vi "GUI_Capillary_Transverse_Diagnostics.vi"() -> ()   [LabVIEW 2020]
uses:
  Shared/GUI_Template/GUI_master/tcp_new_data_event.ctl
  Shared/GUI_Template/GUI_master/tcp new data cluster.ctl
  General GUIs/Device GUIs/GUI_Cameras/color tables/image color table presets.ctl
  <vilib>/Platform/browser.llb/Open URL in Default Browser (string).vi
panel:
  in  "pos.Channel0::6":enum16{"1", "2", "3", "4", "5", "6"}(ring) caption="PL1-PMReflect-FW"
  in  "pos.Channel1::6":enum16{"1", "2", "3", "4", "5", "6"}(ring) caption="PL1-APLSideView FW"
  in  "GUIdevice 6":string="PL1-Filterwheels2"
  in  "Color table":T1=enum."Rainbow"
  in  "GUIdevice 5":string="PL1-SideSpec"
  out "Image::5":T2(plugin-control) caption="PL1-SideSpec"
  in  "GUIdevice 4":string="PL1-PMReflect"
  out "Image::4":T2(plugin-control) caption="PL1-PMReflect"
  in  "GUIdevice 3":string="PL1-SideView"
  out "Image::3":T2(plugin-control) caption="PL1-Sideview"
  in  "GUIdevice 2":string="PL1-APLSideview"
  out "Image::2":T2(plugin-control) caption="PL1-APLSideView"
  out "T/%  810 nm:":dbl
  out "T/%  656 nm:":dbl
  out "T/%  584 nm:":dbl
  out "T/%  532 nm:":dbl
  in  "pos.Channel2::1":enum16{"1", "2", "3", "4", "5", "6"}(ring) caption="PL1-SideSpec-FW"
  out "T/%  810 nm:":dbl
  out "T/%  656 nm:":dbl
  out "T/%  584 nm:":dbl
  out "T/%  532 nm:":dbl
  in  "calc filters":bool
  in  "pos.Channel0::1":enum16{"1", "2", "3", "4", "5", "6"}(ring) caption="PL1-SideView-FW"
  in  "Heater Alignment Directions":bool
  out "error IO 2":errorcluster
  out "tcp data event":T3
  in  "UDP error message":string
  in  "GUIdevice 1":string="PL1-FilterWheels"
  in  "stop":bool
  # "Capillary Monitoring Cameras"
  # "Filter Wheel Overview"
  # "Camera images"
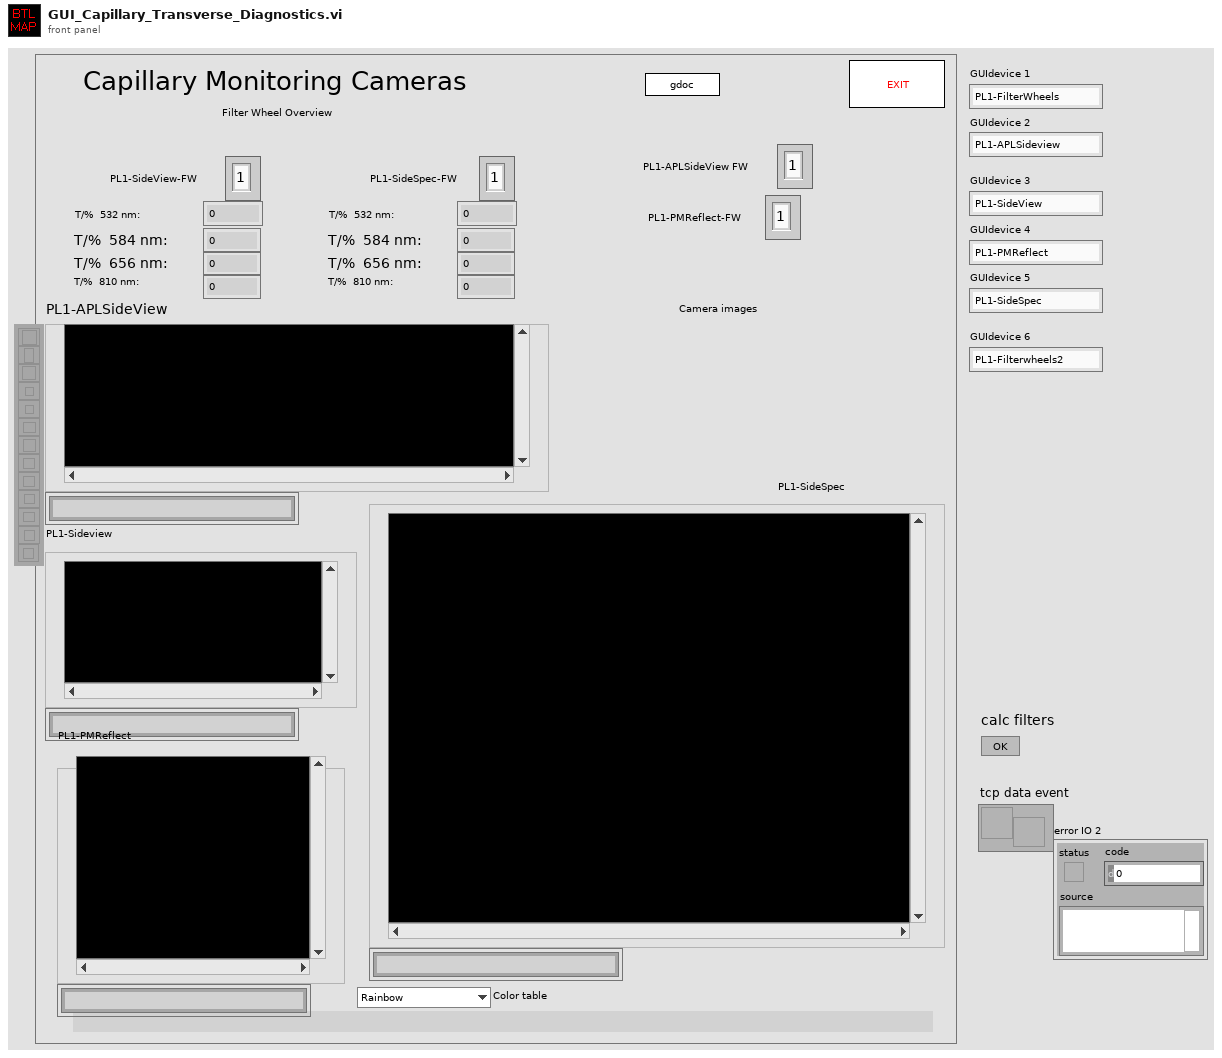
[diagram p1: front panel]
types:
  T1 = typedef "image color table presets.ctl" = enum16{"Greyscale", "Binary", "Gradient", "Rainbow", "Temperature", "enhance low", "blue yellow red", "BYR enhance low", "white blue yellow", "BWR enhance low", "make a new one"}
  T2 = typedef "IMAQ Image.ctl" = refnum<image>
  T3 = typedef "tcp_new_data_event.ctl" = refnum<user-event>
  T4 = typedef "Image Type" = u32
  T5 = typedef "tcp new data cluster.ctl" = cluster{"EventEnum":enum16{"new data", "connection status update"}, "Device name":string}
  T6 = enum32{"invalid app kind", "Development System", "Run Time System", "Student Edition", "Embedded LabVIEW", "Evaluation", "Custom"}
  T7 = enum32{"Invalid", "Standard", "Closed", "Hidden", "Minimized", "Maximized"}
  T8 = cluster{"Core":cluster{"Current VI Reference":refnum<vi>, "Close Panel on Exit?":bool}, "Heater timing offset":dbl, "Discharge timing offset":dbl, "Jet trigger":bool, "Tik1":u32, "Tik2":u32, "Fire Continues Allowed":bool}
  T9 = cluster{"Current VI Reference":refnum<vi>, "Close Panel on Exit?":bool}
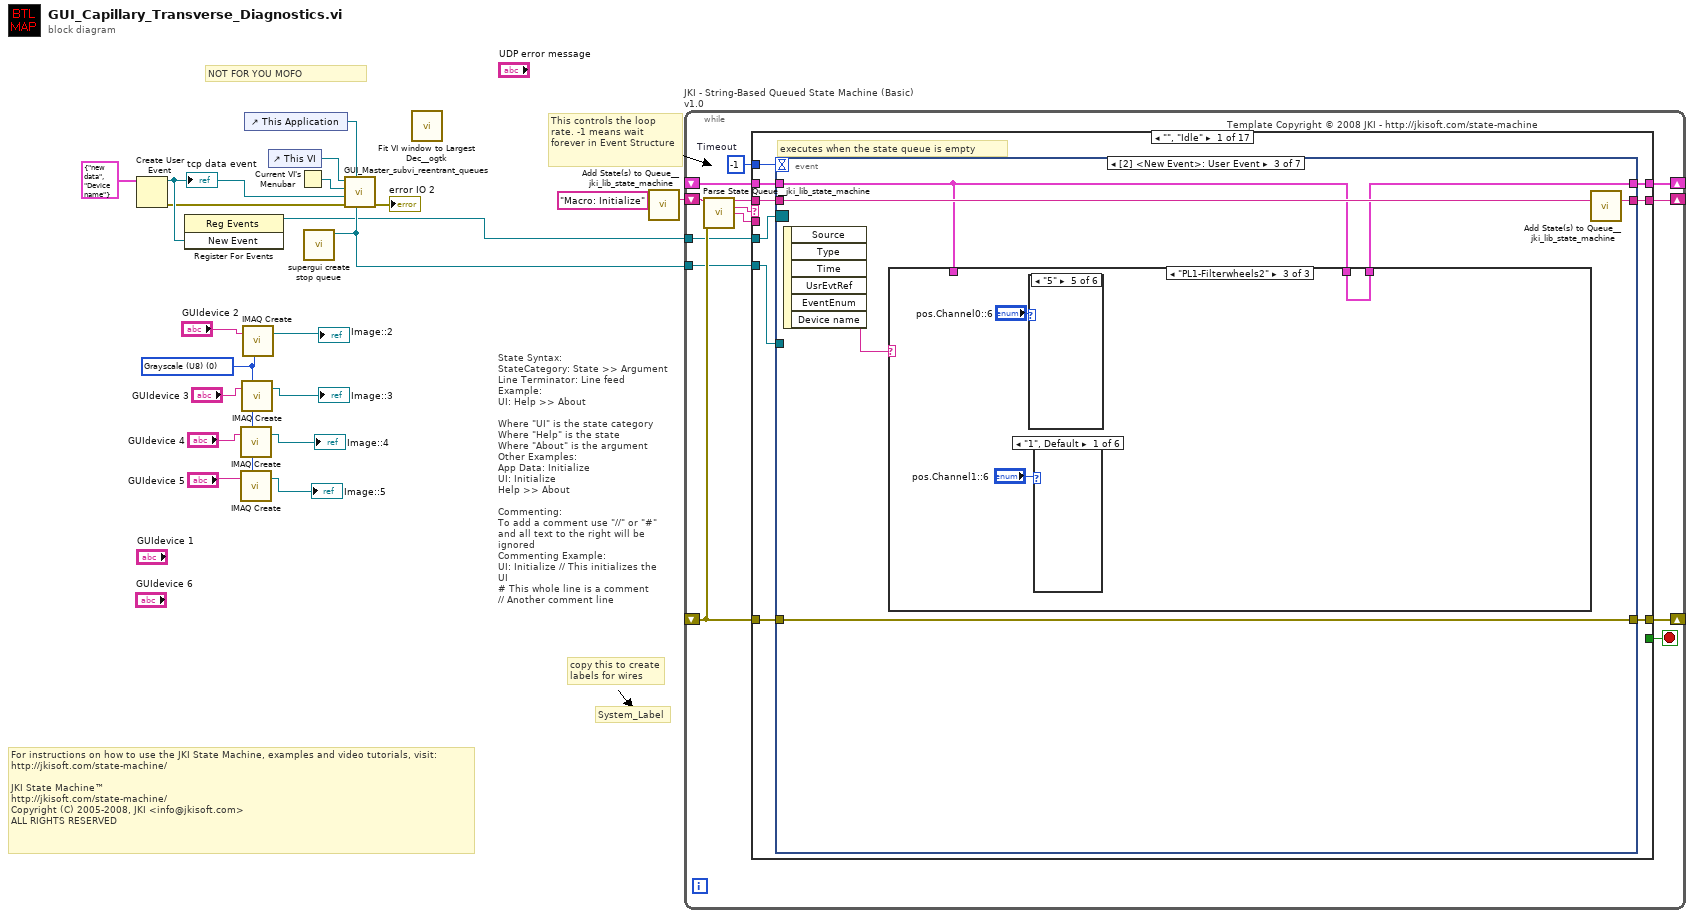
[diagram p0: block diagram]
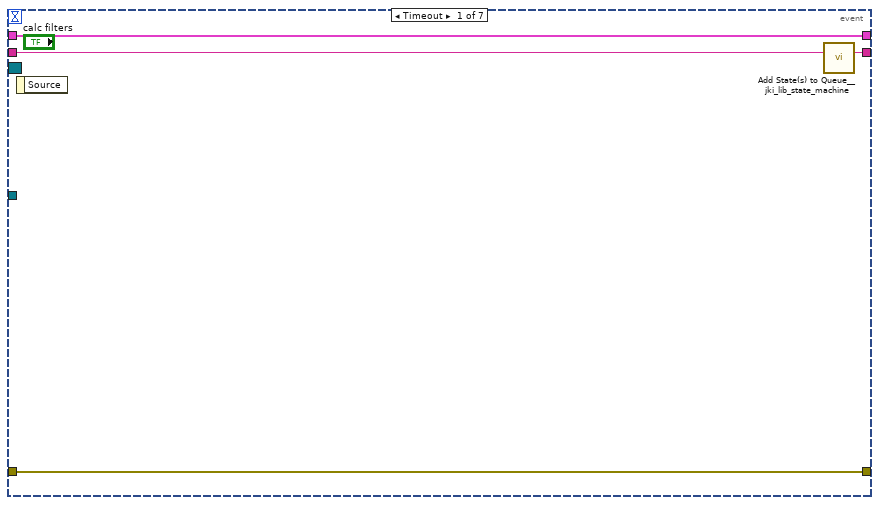
[diagram p2: hidden frame]
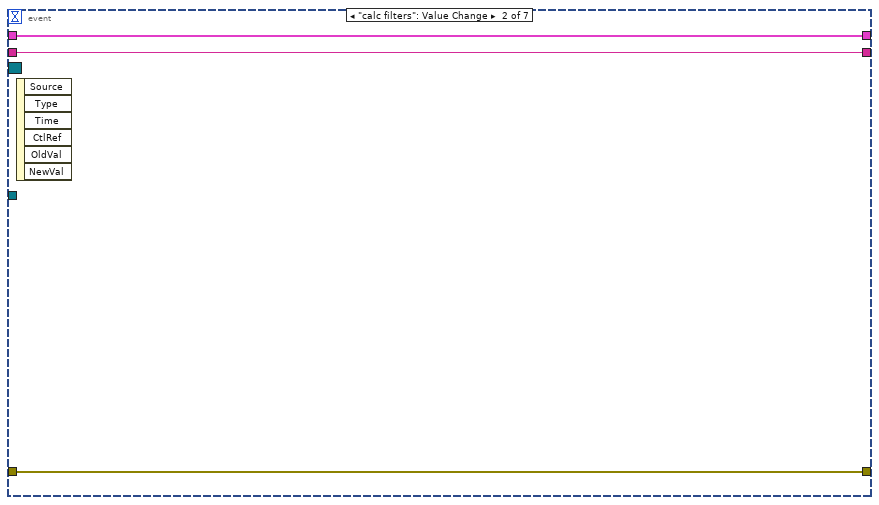
[diagram p3: hidden frame]
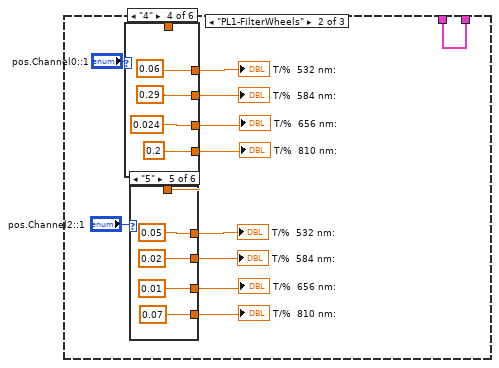
[diagram p5: hidden frame]
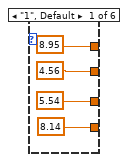
[diagram p6: hidden frame]
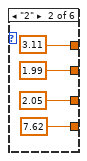
[diagram p7: hidden frame]
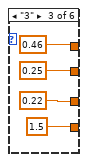
[diagram p8: hidden frame]
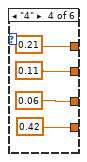
[diagram p9: hidden frame]
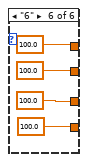
[diagram p10: hidden frame]
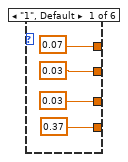
[diagram p11: hidden frame]
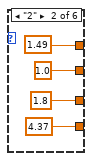
[diagram p12: hidden frame]
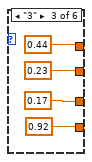
[diagram p13: hidden frame]
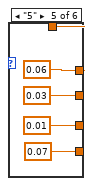
[diagram p14: hidden frame]
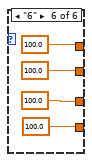
[diagram p15: hidden frame]
diagram:
  w5 = T4 0 items=["Grayscale (U8)", "Grayscale (I16)", "Grayscale (SGL)", "Complex (CSG)", "RGB (U32)", "HSL (U32)", "RGB (U64)", "Grayscale (U16)"] ("Image Type")
  # "For instructions on how to use the JKI State Machine, examples and video tutorials, visit:\nhttp://jkisoft.com/state-machine/\n\nJKI State Machine™\nhttp://jkisoft.com/state-machine/\nCopyright (C) 2005-2008, JKI <info@jkisoft.com>\nALL RIGHTS RESERVED"
  # "State Syntax:\nStateCategory: State >> Argument\nLine Terminator: Line feed\nExample:\nUI: Help >> About\n\nWhere \"UI\" is the state category\nWhere \"Help\" is the state\nWhere \"About\" is the argument\nOther Examples:\nApp Data: Initialize\nUI: Initialize\nHelp >> About\n\nCommenting:\nTo add a comment use \"//\" or \"#\" and all text to the right will be ignored\nCommenting Example:\nUI: Initialize // This initializes the UI\n# This whole line is a comment\n// Another comment line"
  # "copy this to create labels for wires"
  # "This controls the loop rate. -1 means wait forever in Event Structure"
  # "System_Label"
  # "NOT FOR YOU MOFO"
  n1 = Create User Event(user event datatype=T5 {"EventEnum"=enum."new data", "Device name"="Device name"} ("New Event")) -> (user event=w19:refnum<user-event>, error out=w18:errorcluster)  [unwired: 1 in]
  "tcp data event" <- w19
  n2 = register-events(w19) -> (reference out=w10:refnum<event-registration>)  [unwired: 2 in, 1 out]
  n3 = call "IMAQ Create"("Image Name"="GUIdevice 4", "Image Type"=w5) -> ("New Image"=→"Image::4":T2)  [unwired: 3 in, 1 out]
  n4 = call "IMAQ Create"("Image Name"="GUIdevice 5", "Image Type"=w5) -> ("New Image"=→"Image::5":T2)  [unwired: 3 in, 1 out]
  n5 = call "IMAQ Create"("Image Name"="GUIdevice 3", "Image Type"=w5) -> ("New Image"=→"Image::3":T2)  [unwired: 3 in, 1 out]
  n6 = call "IMAQ Create"("Image Name"="GUIdevice 2", "Image Type"=w5) -> ("New Image"=→"Image::2":T2)  [unwired: 3 in, 1 out]
  n7 = control-ref of="This Application"() -> (w20:refnum<vi>)
  n8 = control-ref of="This VI"() -> (w14:refnum<vi>)
  n9 = Current VI's Menubar() -> (w16:refnum<k9>)
  n10 = call "supergui create stop queue.vi"() -> ("STOP Queue out"=w11:refnum<queue>)  [unwired: 11 in]
  n11 = call "GUI_Master_subvi_reentrant_queues.vi"("STOP Queue in"=w11, "This Application"=w20, "error in (no error)"=w18, "tcp data event"=w19, "Caller menu reference"=w16, "Caller VI ref"=w14) -> ("error out"=→"error IO 2":errorcluster)  [unwired: 5 in]
  n12 = call <userlib>:"Fit VI window to Largest Dec__ogtk.vi"() -> ()  [unwired: 6 in, 2 out]
  n13 = call <vilib>:"Add State(s) to Queue__jki_lib_state_machine.vi"("State(s) in (\"\")"="Macro: Initialize") -> ("States Out"=w12:string)  [unwired: 14 in]
  n14 = while "JKI - String-Based Queued State Machine (Basic) v1.0" {
    shift-right: [w26] -> _
    shift-left: _ -> [w25]
    shift-right: [w29] -> _
    shift-left: _ -> [w23]
    shift-right: [w28] -> _
    shift-left: w12 -> [w30]
    tunnel: w10 -> [w22]
    tunnel: w11 -> [w21]
    stop <- w27 stop-if-true
    w24 = -1  # Timeout
    # "Template Copyright © 2008 JKI - http://jkisoft.com/state-machine"
    n15 = call <vilib>:"Parse State Queue__jki_lib_state_machine.vi"("State Queue"=w30, "Error In (no error)"=w23) -> ("Remaining States"=w32:string, "Current State"=w33:string, "Arguments"=w31:string)  [unwired: 11 in]
    n16 = case shown="\"\", \"Idle\"" w33 {
      selector: w33 -> [_ _ w171 _ _ _ _ _ _ _ _ _ _ _ _ _ _]
      tunnel: w32 -> [w42 w170 w175 w193 w199 w204 w208 w219 w225 w229 w235 w241 w252 w278 w283 w293 w297]
      tunnel: w31 -> [_ _ _ _ _ _ _ _ _ _ _ w236 w246 _ _ _ _]
      tunnel: w25 -> [w40 w167 w173 w184 w196 w202 w205 _ w220 w226 w233 w239 w248 w275 w280 w290 w294]
      tunnel: [w39 w168 w177 w190 errorcluster {"status"=FALSE, "code"=0, "source"=""} ("error out") w201 w206 w216 w221 w227 w232 w237 w249 w276 w281 w291 w295] -> w29
      tunnel: w23 -> [w38 w168 w176 w190 w195 w201 w206 w216 w222 w227 w232 w238 w250 w276 w281 w291 w295]
      tunnel: [w41 w169 w174 w192 w198 w203 w207 w218 w224 w228 w234 w240 w251 w277 w282 w292 w296] -> w28
      tunnel: [_ _ _ _ _ TRUE _ _ _ _ _ _ _ _ _ _ _] -> w27
      tunnel: [w34 w167 w173 w191 w196 w202 w205 w217 w220 w226 w233 w239 w248 w275 w280 w290 w294] -> w26
      tunnel: w24 -> [w37 _ _ _ _ _ _ _ _ _ _ _ _ _ _ _ _]
      tunnel: w22 -> [w36 _ _ _ _ _ _ _ _ _ _ _ _ _ _ _ _]
      tunnel: w21 -> [w35 _ _ _ _ _ _ _ _ _ _ _ _ _ _ _ _]
      frame "", "Idle" {
        # "executes when the state queue is empty"
        n17 = event shown="[2] <New Event>: User Event" {
          selector: w36 -> [_ _ _ _ _ _ _]
          dyn-events: _ -> [_ _ _ _ _ _ _]
          timeout: w37 -> [_ _ _ _ _ _ _]
          tunnel: w42 -> [w46 w48 w55 w130 w151 w156 w166]
          tunnel: [w45 w48 w54 w130 w150 w156 w165] -> w41
          tunnel: w40 -> [w43 w49 w51 w131 w148 w155 w163]
          tunnel: [w44 w47 w53 w119 w149 w153 w164] -> w39
          tunnel: w38 -> [w44 w47 w53 w120 w149 w154 w164]
          tunnel: [w43 w49 w50 w131 w148 w155 w163] -> w34
          tunnel: w35 -> [_ _ _ _ w145 _ _]
          event Timeout {
            n18 = event-data() -> ()  [unwired: 1 in, 1 out]
            n19 = call <vilib>:"Add State(s) to Queue__jki_lib_state_machine.vi"("State(s) in (\"\")"=w46) -> ("States Out"=w45:string)  [unwired: 14 in]
          }
          event "calc filters": Value Change {
            n20 = event-data() -> ()  [unwired: 1 in, 6 out]
          }
          event User Event {
            n21 = event-data() -> ("Device name"=w52:string)  [unwired: 1 in, 5 out]
            n22 = case shown="\"PL1-Filterwheels2\"" w52 {
              tunnel: w51 -> [_ _ _]
              tunnel: w51 -> [w56 w67 w118]
              tunnel: [w56 w67 w118] -> w50
              frame "False", Default {
              }
              frame "PL1-FilterWheels" {
                n23 = case shown="\"4\"" "pos.Channel0::1" {
                  tunnel: [_ _ _ _ w111 _] -> _
                  tunnel: [0.07 1.49 0.44 0.06 w111 100.0] -> w66
                  tunnel: [0.03 1.0 0.23 0.29 0.03 100.0] -> w65
                  tunnel: [0.03 1.8 0.17 0.024 0.01 100.0] -> w64
                  tunnel: [0.37 4.37 0.92 0.2 0.07 100.0] -> w63
                  frame "1", Default {
                  }
                  frame "2" {
                  }
                  frame "3" {
                  }
                  frame "4" {
                  }
                  frame "5" {
                    w111 = 0.06
                  }
                  frame "6" {
                  }
                }
                "T/%  532 nm:" <- w66
                "T/%  584 nm:" <- w65
                "T/%  656 nm:" <- w64
                "T/%  810 nm:" <- w63
                n24 = case shown="\"5\"" "pos.Channel2::1" {
                  tunnel: [_ _ _ _ w87 _] -> _
                  tunnel: [8.95 3.11 0.46 0.21 w87 100.0] -> w61
                  tunnel: [4.56 1.99 0.25 0.11 0.02 100.0] -> w60
                  tunnel: [5.54 2.05 0.22 0.06 0.01 100.0] -> w59
                  tunnel: [8.14 7.62 1.5 0.42 0.07 100.0] -> w58
                  frame "1", Default {
                  }
                  frame "2" {
                  }
                  frame "3" {
                  }
                  frame "4" {
                  }
                  frame "5" {
                    w87 = 0.05
                  }
                  frame "6" {
                  }
                }
                "T/%  532 nm:" <- w61
                "T/%  584 nm:" <- w60
                "T/%  656 nm:" <- w59
                "T/%  810 nm:" <- w58
              }
              frame "PL1-Filterwheels2" {
                n25 = case shown="\"5\"" "pos.Channel0::6" {
                  frame "1", Default {
                  }
                  frame "2" {
                  }
                  frame "3" {
                  }
                  frame "4" {
                  }
                  frame "5" {
                  }
                  frame "6" {
                  }
                }
                n26 = case shown="\"1\", Default" "pos.Channel1::6" {
                  frame "1", Default {
                  }
                  frame "2" {
                  }
                  frame "3" {
                  }
                  frame "4" {
                  }
                  frame "5" {
                  }
                  frame "6" {
                  }
                }
              }
            }
            n27 = call <vilib>:"Add State(s) to Queue__jki_lib_state_machine.vi"("State(s) in (\"\")"=w55) -> ("States Out"=w54:string)  [unwired: 14 in]
          }
          event Value Change {
            # "Chech whether user input for color table\nother than Ni pallete"
            # "When user cancels the make new one color table \nthen color table value changed to rainbow"
            n28 = event-data() -> ()  [unwired: 1 in, 6 out]
            n29 = control-ref of="Image::4"() -> (w121:refnum<vi>)
            n30 = property on="Color table" class="Enum (strict)"() -> ("Strings []"=w125:string[])  [unwired: 2 in, 2 out]
            n31 = Format Into String("Color table") -> (resulting string=w124:string)  [unwired: 3 in, 1 out]
            n32 = call "IMAQ color table presets.vi"("Color table"="Color table") -> ("Make new one cancelled"=w129:bool, "Array"=w122:cluster{"R":u8, "G":u8, "B":u8}[])  [unwired: 9 in]
            n33 = Search 1D Array(1D array=w125, element=w124) -> (index of element=w127:i32)  [unwired: 1 in]
            n34 = Greater Or Equal?(x=w127, y=5) -> (x >= y?=w126:bool)
            n35 = case shown="False" w126 {
              tunnel: w122 -> [_ w140]
              tunnel: "Color table" -> [w135 _]
              tunnel: w120 -> [w134 w137]
              tunnel: [w133 w139] -> w119
              tunnel: w129 -> [_ w138]
              tunnel: w121 -> [w132 w136]
              frame False {
                n36 = property on="Property Node" class="ImageControl"(reference=w132, error in=w134, "Palette Type"=w135) -> (error out=w133:errorcluster)  [unwired: 1 out]
              }
              frame True {
                w141 = u32 5 items=["Grayscale", "Binary", "Gradient", "Rainbow", "Temperature", "User Defined"] ("Palette:Palette Type")
                n37 = property on="Property Node" class="ImageControl"(reference=w136, error in=w137, "Palette Type"=w141, "User Palette"=w140) -> (error out=w139:errorcluster)  [unwired: 1 out]
                n38 = case shown="True" w138 {
                  tunnel: w137 -> [_ w142]
                  frame False {
                  }
                  frame True {
                    n39 = property on="Color table" class="Enum (strict)"(error in=w142, "Val(Sgnl)"=image_color_table_presets."Rainbow" ("Value (Signaling)")) -> ()  [unwired: 1 in, 2 out]
                  }
                }
              }
            }
          }
          event "stop": Value Change {
            # "Exit Button Value Change (pressed) Event\n(this executes Macro: Exit to terminate the VI)"
            n40 = event-data() -> ()  [unwired: 1 in, 6 out]
            n41 = Release Queue(queue=w145, force destroy? (F)=TRUE) -> (error out=w146:errorcluster)  [unwired: 1 in, 2 out]
            n42 = call <vilib>:"Clear Errors.vi"("error in (no error)"=w146) -> ()  [unwired: 5 in, 2 out]
            n43 = call <vilib>:"Add State(s) to Queue__jki_lib_state_machine.vi"("State(s) in Front (\"\")"="Macro: Exit", "State(s) in (\"\")"=w151) -> ("States Out"=w150:string)  [unwired: 13 in]
          }
          event "Heater Alignment Directions": Value Change {
            n44 = event-data() -> ()  [unwired: 1 in, 6 out]
            n45 = case shown="True" "Heater Alignment Directions" {
              tunnel: w154 -> [w157 w160]
              tunnel: [w157 w159] -> w153
              frame False {
              }
              frame True {
                n46 = call-poly <vilib>:"Open URL in Default Browser.vi"("error in (no error)"=w160, "URL"="https://docs.google.com/document/d/11rq5sV6otXhl_RvgO5tmtLmhp9iuGuESqiH9zh7F1jg/edit?usp=sharing") -> ("error out"=w159:errorcluster)  [unwired: 4 in, 1 out]
              }
            }
          }
          event Panel Close? {
            # "Discard the event because we'll close the front panel ourselves in Macro: Exit"
            # "Close Panel button (pressed) Event\n(this executes Macro: Exit to terminate the VI)"
            n47 = event-data() -> ()  [unwired: 1 in, 1 out]
            n48 = event-data("Discard?"=TRUE) -> ()  [unwired: 1 in, 1 out]
            n49 = call <vilib>:"Add State(s) to Queue__jki_lib_state_machine.vi"("State(s) in Front (\"\")"="Macro: Exit", "State(s) in (\"\")"=w166) -> ("States Out"=w165:string)  [unwired: 13 in]
          }
        }
      }
      frame "---------- Core ----------" {
        # "Do not put any code in this frame.\n(it is a separator no-op)"
        n50 = call <vilib>:"Add State(s) to Queue__jki_lib_state_machine.vi"("State(s) in (\"\")"=w170) -> ("States Out"=w169:string)  [unwired: 14 in]
      }
      frame Default {
        w180 = 42 items=["No error", "Argument error", "Memory is full", "Out of zone", "End of file", "File already open", "Generic file I/O error", "File not found", "File permission error", "Disk is full", "Duplicate path", "Too many files open", "System feature not enabled", "Resource file not found", "Cannot add resource", "Resource not found", "Image not found", "Image memory error", "Pen does not exist", "Config type invalid", "Config token not found", "Config parse error", "Config memory error", "Bad external code format", "Bad external code offset", "External code not present", "Null window", "Destroy window error", "Null menu", "Print aborted", "Bad print record", "Print driver error", "Windows error during printing", "Memory error during printing", "Print dialog error", "Generic print error", "Invalid device refnum", "Device not found", "Device parameter error", "Device unit error", "Cannot open device", "Device call aborted", "Generic error", "Cancelled by user", "Object ID too low", "Object ID too high", "Object not in heap", "Unknown heap", "Unknown object (invalid DefProc)", "Unknown object (DefProc not in table)", "Message out of range", "Invalid (null) method", "Unknown message", "Manager call not supported", "Bad address", "Network operation in progress", "Network operation timed out", "Connection is busy", "Network attribute not supported", "Network error", "Address in use", "System out of memory", "Connection aborted", "Connection refused", "Not connected", "Already connected", "Connection closed", "Initialization error (interapplication manager)", "Bad occurrence", "Wait on unbound occurrence handler", "Occurrence queue overflow", "Datalog type conflict", "Unused", "Unrecognized type (interapplication manager)", "Memory corrupt", "Failed to make temporary DLL", "Old CIN version", "Drag socket not found", "Failed to load drop-object", "Failed to register OLE object", "Failed to release OLE object", "Format specifier type mismatch", "Unknown format specifier", "Too few format specifiers", "Too many format specifiers", "Scan failed", "Newer CIN version", "Error converting to variant", "Runtime menu error", "Password tampered", "Variant attribute not found", "Incompatible variant data type", "Event data is not available", "Event Store is not present", "Occurrence is not found", "Event Queue is not created", "Event info is not available", "Refnum passed is NULL", "Error retrieving Class GUID", "Error retrieving CoClass GUID", "Error retrieving TypeLib GUID.", "Bad built application magic bytes.", "Specific driver is different from the specific driver associated with the Logical Name.", "There is no session opened to the class driver.", "Max Error", "MAX - Error with config objects", "MAX - Error loading configuration", "MAX - Group not supported"]
        # "Current State"
        # "Do not delete, rename, or modify this frame.\n(this is used to capture unhandled states and typos)"
        # "Handle mistyped state name (developer tool)"
        n51 = Format Into String(format string="Software Exception: Unhandled State \"%s\"." ("message"), error in=w176, w171) -> (resulting string=w179:string, error out=w178:errorcluster)  [unwired: 1 in]
        n52 = call <vilib>:"Error Cluster From Error Code.vi"("show call chain? (False)"=TRUE, "error in (no error)"=w178, "error message (\"\")"=w179, "error code (0)"=w180) -> ("error out"=w177:errorcluster)  [unwired: 5 in]
        n53 = call <vilib>:"Add State(s) to Queue__jki_lib_state_machine.vi"("State(s) in (\"\")"=w175) -> ("States Out"=w174:string)  [unwired: 14 in]
      }
      frame "Initialize Core Data" {
        # "Do not delete, rename, or modify this frame.\n(this is used to determine panel behavior on exit)"
        # "originally closed?"
        # "exe?"
        # "If panel starts closed or is an EXE, then close it when we exit"
        n54 = property class="VI"() -> ("Front Panel.Open"=w189:bool)  [unwired: 2 in, 2 out]
        n55 = property class="App"() -> ("App.Kind"=w188:T6)  [unwired: 2 in, 2 out]
        n56 = control-ref of="Current VI Reference"() -> (w182:refnum<vi>)
        n57 = Not(x=w189) -> (.not. x?=w186:bool)
        n58 = Equal?(x=w188, y=T6."Run Time System" ("Application:Kind")) -> (x = y?=w185:bool)
        n59 = Or(x=w186, y=w185) -> (x .or. y?=w183:bool)
        n60 = Bundle By Name(cluster=w184, "Core.Current VI Reference"=w182, "Core.Close Panel on Exit?"=w183) -> (w191:T8)
        n61 = call <vilib>:"Add State(s) to Queue__jki_lib_state_machine.vi"("State(s) in (\"\")"=w193) -> ("States Out"=w192:string)  [unwired: 14 in]
      }
      frame "Error Handler" {
        # "Unhandled Error -- Display it"
        # "Handle any errors here.\nYou can also output any states to clean-up after errors occur"
        # "Clear error"
        n62 = call <vilib>:"General Error Handler.vi"("error in (no error)"=w195) -> ()  [unwired: 10 in, 5 out]
        n63 = call <vilib>:"Add State(s) to Queue__jki_lib_state_machine.vi"("State(s) in Front (\"\")"="/* Post Error States", "State(s) in (\"\")"=w199) -> ("States Out"=w198:string)  [unwired: 13 in]
      }
      frame "Exit" {
        # "Do not put any code in this frame.\n(No errors that occur here will be handled.)"
        n64 = call <vilib>:"Add State(s) to Queue__jki_lib_state_machine.vi"("State(s) in (\"\")"=w204) -> ("States Out"=w203:string)  [unwired: 14 in]
      }
      frame "---------- Data ----------" {
        # "Do not put any code in this frame.\n(It is a separator no-op. You can make a copy of this frame to create a new Data frame)"
        n65 = call <vilib>:"Add State(s) to Queue__jki_lib_state_machine.vi"("State(s) in (\"\")"=w208) -> ("States Out"=w207:string)  [unwired: 14 in]
      }
      frame "Data: Initialize" {
        w209 = FALSE  # Fire Continues Allowed
        w211 = u32 0  # Tik1
        w210 = u32 0  # Tik2
        w212 = FALSE  # Jet trigger
        w213 = 0.0  # Discharge timing offset
        w214 = 0.0  # Heater timing offset
        w215 = T9 {"Current VI Reference"=refnum, "Close Panel on Exit?"=FALSE}  # Core
        # "do not delete - used by framework"
        # "Expand Bundle to add new data elements to shift register data."
        # "Add new data here."
        # "Data names and types of shift register data are defined by this bundle."
        # "Initialize the shift-register data, here.\n(data names are defined by what you wire into the bundle function)"
        n66 = Bundle("Core"=w215, "Heater timing offset"=w214, "Discharge timing offset"=w213, "Jet trigger"=w212, "Tik1"=w211, "Tik2"=w210, "Fire Continues Allowed"=w209) -> (w217:T8)  [unwired: 1 in]
        n67 = call <vilib>:"Add State(s) to Queue__jki_lib_state_machine.vi"("State(s) in (\"\")"=w219) -> ("States Out"=w218:string)  [unwired: 14 in]
      }
      frame "Data: Cleanup" {
        # "Cleanup any data and references, here.\n(this is called automatically, by the Macro: Exit)"
        n68 = Unbundle By Name(w220) -> ("Core.Current VI Reference"=w223:refnum<vi>)
        n69 = Close Reference(reference=w223, error in (no error)=w222) -> (error out=w221:errorcluster)
        n70 = call <vilib>:"Add State(s) to Queue__jki_lib_state_machine.vi"("State(s) in (\"\")"=w225) -> ("States Out"=w224:string)  [unwired: 14 in]
      }
      frame "---------- UI ----------" {
        # "Do not put any code in this frame.\n(It is a separator no-op. You can make a copy of this frame to create a new UI frame)"
        n71 = call <vilib>:"Add State(s) to Queue__jki_lib_state_machine.vi"("State(s) in (\"\")"=w229) -> ("States Out"=w228:string)  [unwired: 14 in]
      }
      frame "UI: Initialize" {
        # "Initialize the User Interface, here.\n(this is called automatically, by the Macro: Init)"
        n72 = control-ref of="Color table"() -> (w230:refnum<vi>)
        n73 = property on="Property Node" class="Enum (strict)"(reference=w230, "Value"=image_color_table_presets."Rainbow" ("Color table")) -> ()  [unwired: 1 in, 2 out]
        n74 = call <vilib>:"Add State(s) to Queue__jki_lib_state_machine.vi"("State(s) in (\"\")"=w235) -> ("States Out"=w234:string)  [unwired: 14 in]
      }
      frame "UI: Cursor Set" {
        # "Argument"
        # "Set and Unset Cursor Busy.\n(Usage: \"UI: Cursor Set >> Busy|Idle\")"
        n75 = case shown="\"Idle\", Default" w236 {
          tunnel: w238 -> [w243 w245]
          tunnel: [w242 w244] -> w237
          frame "Idle", Default {
            n76 = call <vilib>:"Unset Busy.vi"("error in (no error)"=w243) -> ("error out"=w242:errorcluster)  [unwired: 10 in]
          }
          frame "Busy" {
            n77 = call <vilib>:"Set Busy.vi"("error in (no error)"=w245) -> ("error out"=w244:errorcluster)  [unwired: 9 in, 1 out]
          }
        }
        n78 = call <vilib>:"Add State(s) to Queue__jki_lib_state_machine.vi"("State(s) in (\"\")"=w241) -> ("States Out"=w240:string)  [unwired: 14 in]
      }
      frame "UI: Front Panel State" {
        # "Argument"
        # "Set Front Panel Open or Closed\n(Usage: \"UI: Front Panel State >> Open|Close\")"
        n79 = Unbundle By Name(w248) -> ("Core.Current VI Reference"=w247:refnum<vi>)
        n80 = case shown="\"Close\"" w246 {
          tunnel: w250 -> [w256 w269]
          tunnel: [w258 w270] -> w249
          tunnel: w247 -> [w257 w267]
          frame "Open", Default {
            n81 = property class="VI"(reference=w257, error in=w256) -> (reference out=w254:refnum<vi>, error out=w255:errorcluster, "Front Panel.Open"=w253:bool)
            n82 = case shown="False" w253 {
              tunnel: [w261 w264] -> w258
              tunnel: w255 -> [w260 w264]
              tunnel: w254 -> [w259 _]
              frame False {
                n83 = invoke class="VI" method="FP.Open"(reference=w259, error in=w260, "Activate"=TRUE, "State"=T7."Standard") -> (error out=w261:errorcluster)  [unwired: 1 in, 4 out]
              }
              frame True {
              }
            }
          }
          frame "Close" {
            n84 = property class="VI"(reference=w267, error in=w269) -> (reference out=w266:refnum<vi>, error out=w268:errorcluster, "Front Panel.Open"=w265:bool)
            n85 = case shown="True" w265 {
              tunnel: [w271 w274] -> w270
              tunnel: w268 -> [w271 w273]
              tunnel: w266 -> [_ w272]
              frame False {
              }
              frame True {
                n86 = invoke class="VI" method="FP.Close"(reference=w272, error in=w273) -> (error out=w274:errorcluster)  [unwired: 1 in, 2 out]
              }
            }
          }
        }
        n87 = call <vilib>:"Add State(s) to Queue__jki_lib_state_machine.vi"("State(s) in (\"\")"=w252) -> ("States Out"=w251:string)  [unwired: 14 in]
      }
      frame "---------- Macro ----------" {
        # "Do not put any code in this frame.\n(It is a separator no-op. You can make a copy of this frame to create a new Macro frame)"
        n88 = call <vilib>:"Add State(s) to Queue__jki_lib_state_machine.vi"("State(s) in (\"\")"=w278) -> ("States Out"=w277:string)  [unwired: 14 in]
      }
      frame "Macro: Initialize" {
        w279 = "Data: Initialize\nInitialize Core Data\nUI: Initialize\nUI: Front Panel State >> Open"  # Data: Initialize Initialize Core Data UI: Initialize UI: Front Panel State >> Open
        # "Initialization Macro\n(This is called once, when the VI starts)"
        n89 = call <vilib>:"Add State(s) to Queue__jki_lib_state_machine.vi"("State(s) in Front (\"\")"=w279, "State(s) in (\"\")"=w283) -> ("States Out"=w282:string)  [unwired: 13 in]
      }
      frame "Macro: Exit" {
        # "Exit Macro\n(This is called once, when the VI exits)"
        n90 = Unbundle By Name(w290) -> ("Core.Close Panel on Exit?"=w289:bool)
        n91 = Select(t="UI: Front Panel State >> Close", s=w289, f="") -> (s? t:f=w286:string)
        n92 = call <vilib>:"Add State(s) to Queue__jki_lib_state_machine.vi"("State(s) in (\"\")"=w286, "State(s) at Back (\"\")"="Data: Cleanup\nExit") -> ("States Out"=w284:string)  [unwired: 13 in]
        n93 = call <vilib>:"Add State(s) to Queue__jki_lib_state_machine.vi"("State(s) in Front (\"\")"=w284, "State(s) in (\"\")"=w293) -> ("States Out"=w292:string)  [unwired: 13 in]
      }
      frame "---------- New Category ----------" {
        # "Template Separator\n(You can make a copy of, or modify, this frame)"
        n94 = call <vilib>:"Add State(s) to Queue__jki_lib_state_machine.vi"("State(s) in (\"\")"=w297) -> ("States Out"=w296:string)  [unwired: 14 in]
      }
    }
  }
